vi "CALC_SMO_APER.vi"(0 "VISA IN":refnum<visa-resource-name>, 1 "Percentage Value":i32, 5 "error in":errorcluster, 7 "Channel":i32) -> (14 "VISA Out":refnum<visa-resource-name>, 19 "error out":errorcluster)   [LabVIEW 2018, in "PNA-X.lvlib"]
doc: "CALCulate<cnum>:SMOothing:APERture <num> \n(Read-Write) Sets the amount of smoothing as a percentage of the number of data points in the \nchannel. \nSee Critical Note \nParameters \n<cnum> Channel number of the measurement. There must be a selected measurement \non that channel. If unspecified, <cnum> is set to 1. \n<num> Percentage value. Choose any number between: \n1 and 25 \nExamples CALC:SMO:APER 2 \ncalculate2:smoothing:aperture 20.7 \nQuery Syntax CALCulate<cnum>:SMOothing:APERture? \nReturn Type Numeric \n1563\n\nDefault 1.5"
uses:
  PNA-X.lvlib
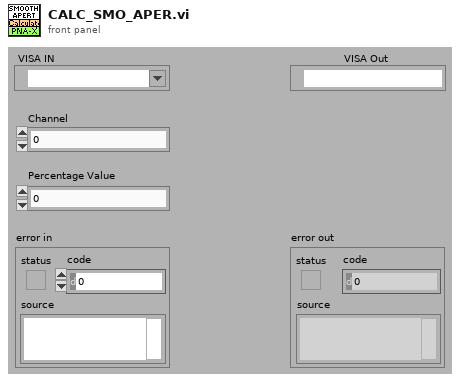
[diagram p1: front panel]
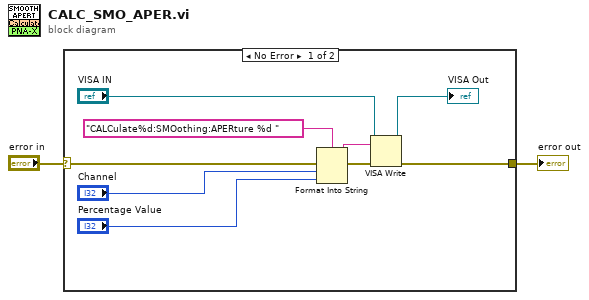
[diagram p0: block diagram]
diagram:
  n1 = case shown="No Error" "error in" {
    selector: "error in" -> [w11 w12]
    tunnel: [w6 w12] -> w1
    frame No Error {
      n2 = Format Into String(format string="CALCulate%d:SMOothing:APERture %d " ("Cmdline"), error in=w11, "Channel", "Percentage Value") -> (resulting string=w9:string, error out=w10:errorcluster)  [unwired: 1 in]
      n3 = VISA Write(VISA resource name="VISA IN", write buffer=w9, error in (no error)=w10) -> (VISA resource name out=→"VISA Out":refnum<visa-resource-name>, error out=w6:errorcluster)  [unwired: 1 out]
    }
    frame Error {
    }
  }
  "error out" <- w1
